vi "SaveSpeedProfileData.vi"(6 "registry":T16, 7 "data event data":T1, 8 "error in (no error)":errorcluster, 10 "pulse positions array":T9[](array[typedef]), 11 "data event config":T10) -> (0 "error out":errorcluster, 3 "data event data out":T1)   [LabVIEW 2017, in "CmsDataEventCreator.lvlib"]
uses:
  <vilib>/addons/InsightCM/Devices/Shared/Cms/CmsDataEventCreator/CmsDataEventCreator.lvlib
  <vilib>/addons/InsightCM/Devices/Shared/Cms/CmsDataEventCreator/controls/GroupRegistry.ctl
  <vilib>/addons/InsightCM/Devices/Shared/Cms/CmsDataEventCreator/controls/DataSetRegistry.ctl
  <vilib>/addons/InsightCM/Devices/Shared/Common/DataEvent/controls/DataSetType.ctl
  <vilib>/addons/InsightCM/Devices/Shared/Common/DataEventCreator/controls/Registry_Trend.ctl
  <vilib>/addons/InsightCM/Devices/Shared/Cms/CmsDataEventCreator/controls/DataEventConfig.ctl
  <vilib>/addons/InsightCM/Devices/Shared/Cms/CmsDataEventCreator/controls/AcqParams.ctl
  <vilib>/addons/InsightCM/Devices/Shared/Common/DataAccumulator/controls/AccumulationSettings.ctl
  <vilib>/addons/InsightCM/Devices/Shared/Common/DataAccumulator/controls/accumulationType.ctl
  <vilib>/addons/InsightCM/Devices/Shared/Common/DVRBuffer/controls/BufferLocation.ctl
  <vilib>/addons/PointValueMap/controls/PointMap.ctl
  <vilib>/addons/InsightCM/Utilities/Analysis/Shared/controls/PulsePositions.ctl
  <vilib>/addons/InsightCM/Devices/Shared/Common/DataEvent/controls/Event.ctl
  <vilib>/addons/InsightCM/MessageBus/Base/controls/DataEvent.ctl
  <vilib>/addons/InsightCM/MessageBus/Base/controls/KeyValuePair.ctl
  <vilib>/addons/InsightCM/Devices/Shared/Common/DataEvent/controls/DataSet.ctl
  <vilib>/addons/InsightCM/MessageBus/Base/controls/DataSetMetadata.ctl
  <vilib>/addons/InsightCM/MessageBus/Base/controls/TrendPoint.ctl
  <vilib>/addons/InsightCM/MessageBus/Base/controls/TrendAlarmUpdate.ctl
  <vilib>/addons/InsightCM/MessageBus/Base/controls/TrendAlarmTransition.ctl
  <vilib>/addons/PointValueMap/PointValueMap.lvlib
  <vilib>/addons/InsightCM/Devices/Shared/Common/DataEvent/DataEvent.lvlib
  <vilib>/addons/InsightCM/Devices/Shared/Common/DataEventCreator/DataEventCreator.lvlib
  <vilib>/addons/InsightCM/Devices/Shared/Common/DataAccumulator/DataAccumulator.lvlib
  <vilib>/addons/InsightCM/Devices/Shared/Common/DVRBuffer/DVRBuffer.lvlib
  <vilib>/addons/InsightCM/Utilities/Analysis/Shared/AnalysisHelper.lvlib
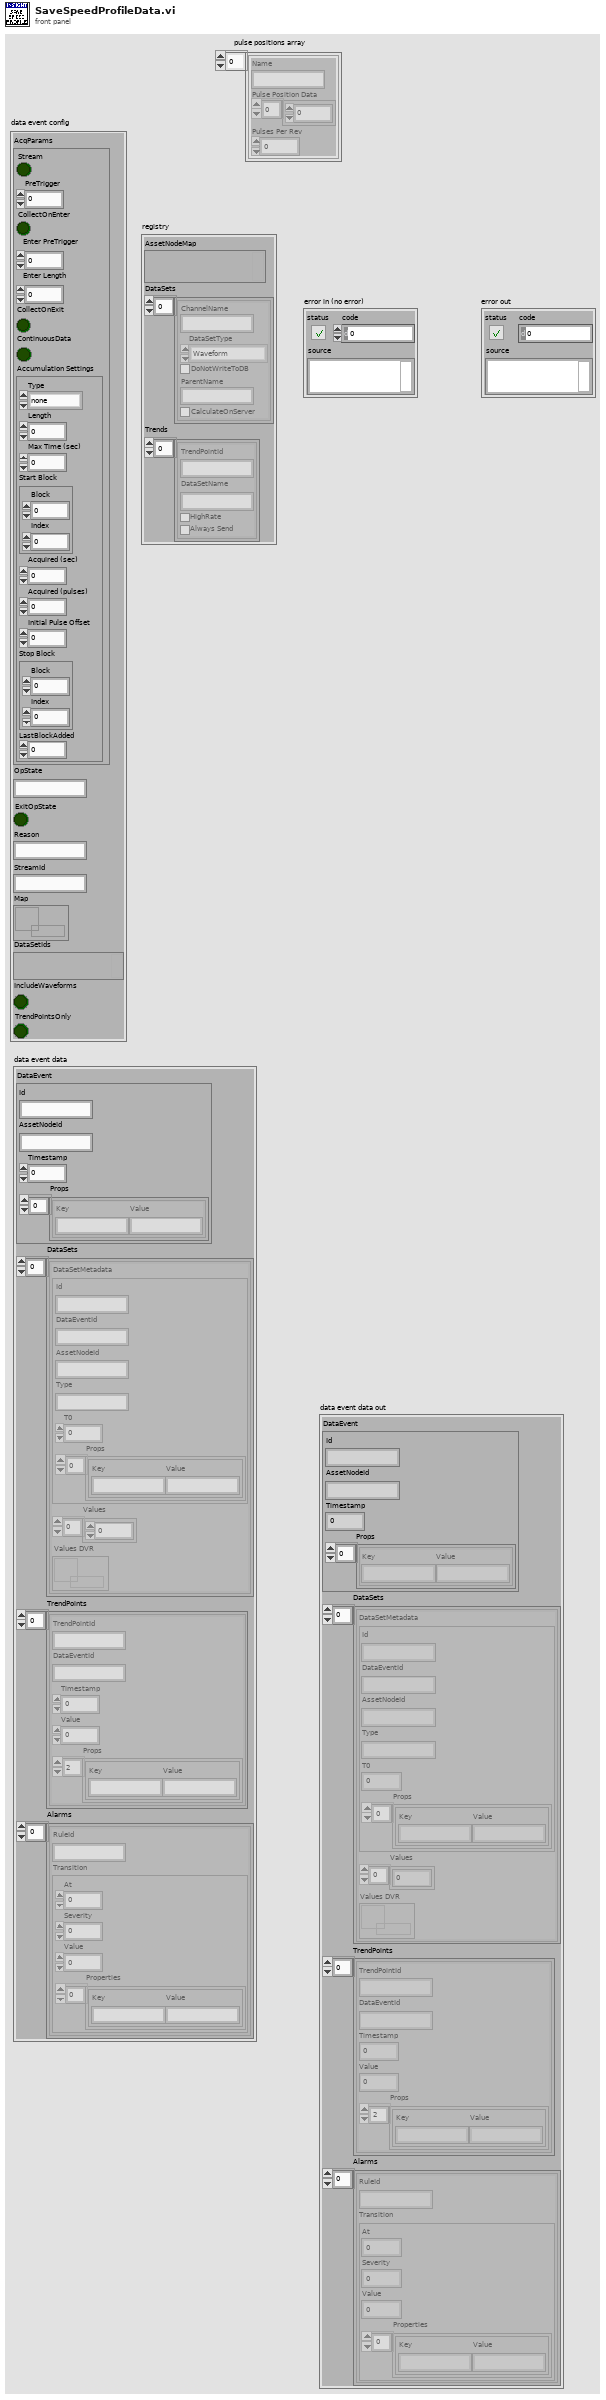
[diagram p1: front panel]
types:
  T1 = typedef "DataEvent.lvlib/Event.ctl" = cluster{"DataEvent":T2, "DataSets":T4[], "TrendPoints":T6[], "Alarms":T7[]}
  T2 = typedef "DataEvent.ctl" = cluster{"Id":string, "AssetNodeId":string, "Timestamp":i64, "Props":T3[]}
  T3 = typedef "KeyValuePair.ctl" = cluster{"Key":string, "Value":string}
  T4 = typedef "DataEvent.lvlib/DataSet.ctl" = cluster{"DataSetMetadata":T5, "Values":sgl[], "Values DVR":refnum<data-value>}
  T5 = typedef "DataSetMetadata.ctl" = cluster{"Id":string, "DataEventId":string, "AssetNodeId":string, "Type":string, "T0":i64, "Props":T3[]}
  T6 = typedef "TrendPoint.ctl" = cluster{"TrendPointId":string, "DataEventId":string, "Timestamp":i64, "Value":dbl, "Props":T3[]}
  T7 = typedef "TrendAlarmUpdate.ctl" = cluster{"RuleId":string, "Transition":T8}
  T8 = typedef "TrendAlarmTransition.ctl" = cluster{"At":i64, "Severity":i32, "Value":dbl, "Properties":T3[]}
  T9 = typedef "AnalysisHelper.lvlib/PulsePositions.ctl" = cluster{"Name":string, "Pulse Position Data":dbl[], "Pulses Per Rev":i32}
  T10 = typedef "CmsDataEventCreator.lvlib/DataEventConfig.ctl" = cluster{"AcqParams":T11, "OpState":string, "ExitOpState":bool, "Reason":string, "StreamId":string, "Map":T15, "DataSetIds":variant, "IncludeWaveforms":bool, "TrendPointsOnly":bool}
  T11 = typedef "CmsDataEventCreator.lvlib/AcqParams.ctl" = cluster{"Stream":bool, "PreTrigger":i32, "CollectOnEnter":bool, "Enter PreTrigger":i32, "Enter Length":dbl, "CollectOnExit":bool, "ContinuousData":bool, "Accumulation Settings":T12}
  T12 = typedef "DataAccumulator.lvlib/AccumulationSettings.ctl" = cluster{"Type":T13, "Length":dbl, "Max Time (sec)":dbl, "Start Block":T14, "Acquired (sec)":dbl, "Acquired (pulses)":i32, "Initial Pulse Offset":dbl, "Stop Block":T14, "LastBlockAdded":u32}
  T13 = typedef "DataAccumulator.lvlib/accumulationType.ctl" = enum16{"none", "seconds", "revolutions"}
  T14 = typedef "DVRBuffer.lvlib/BufferLocation.ctl" = cluster{"Block":u32, "Index":i32}
  T15 = typedef "PointValueMap.lvlib/PointMap.ctl" = refnum<data-value>
  T16 = typedef "CmsDataEventCreator.lvlib/GroupRegistry.ctl" = cluster{"AssetNodeMap":variant, "DataSets":T17[], "Trends":T19[]}
  T17 = typedef "CmsDataEventCreator.lvlib/DataSetRegistry.ctl" = cluster{"ChannelName":string, "DataSetType":T18, "DoNotWriteToDB":bool, "ParentName":string, "CalculateOnServer":bool}
  T18 = typedef "DataEvent.lvlib/DataSetType.ctl" = enum16{"Waveform", "SpeedProfile", "ThermalImage", "EmsaSweep"}
  T19 = typedef "DataEventCreator.lvlib/Registry_Trend.ctl" = cluster{"TrendPointId":string, "DataSetName":string, "HighRate":bool, "Always Send":bool}
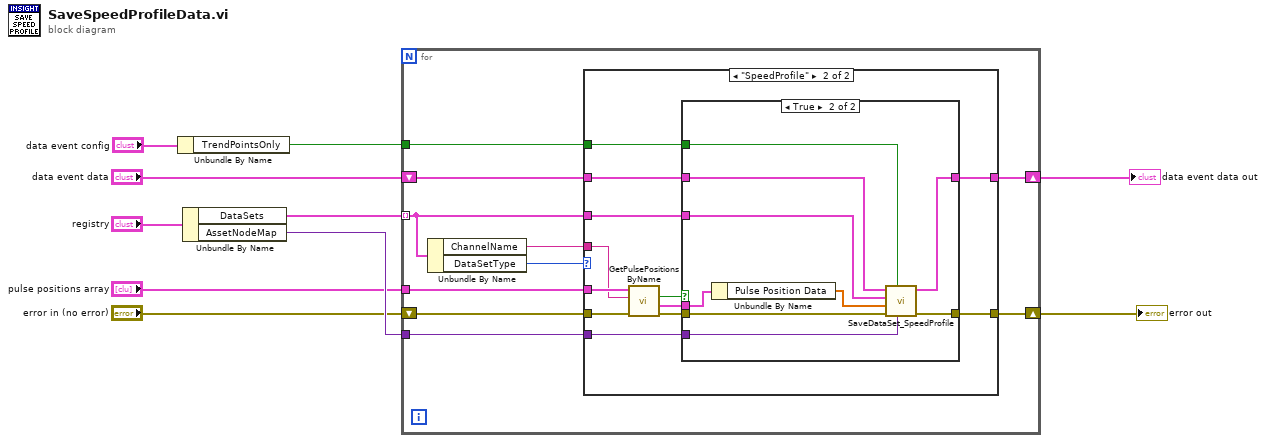
[diagram p0: block diagram]
diagram:
  n1 = Unbundle By Name("data event config") -> ("TrendPointsOnly"=w3:bool)
  n2 = Unbundle By Name("registry") -> ("DataSets"=w9:T17[], "AssetNodeMap"=w6:variant)
  n3 = for {
    tunnel: w9 -> [w13] mode=indexing
    shift-right: [w20] -> w8
    shift-left: "error in (no error)" -> [w19]
    shift-right: [w16] -> w1
    shift-left: "data event data" -> [w18]
    tunnel: "pulse positions array" -> [w15]
    tunnel: w6 -> [w12]
    tunnel: w3 -> [w11]
    n4 = Unbundle By Name(w13) -> ("ChannelName"=w17:string, "DataSetType"=w14:T18)
    n5 = case shown="\"SpeedProfile\"" w14 {
      tunnel: [w22 w34] -> w20
      tunnel: w19 -> [w22 w33]
      tunnel: w18 -> [w21 w32]
      tunnel: w17 -> [_ w26]
      tunnel: [w21 w31] -> w16
      tunnel: w15 -> [_ w30]
      tunnel: w13 -> [_ w25]
      tunnel: w12 -> [_ w24]
      tunnel: w11 -> [_ w23]
      frame Default {
      }
      frame "SpeedProfile" {
        n6 = call <vilib>:"GetPulsePositionsByName.vi"("error in (no error)"=w33, "Channel Name"=w26, "Pulse Positions Array"=w30) -> ("error out"=w29:errorcluster, "Pulse Positions"=w28:T9, "Found?"=w27:bool)  [unwired: 5 in, 1 out]
        n7 = case shown="True" w27 {
          tunnel: [w35 w44] -> w34
          tunnel: w32 -> [w36 w43]
          tunnel: [w36 w42] -> w31
          tunnel: w29 -> [w35 w45]
          tunnel: w28 -> [_ w39]
          tunnel: w25 -> [_ w41]
          tunnel: w24 -> [_ w40]
          tunnel: w23 -> [_ w37]
          frame False {
          }
          frame True {
            n8 = Unbundle By Name(w39) -> ("Pulse Position Data"=w38:dbl[])
            n9 = call <vilib>:"SaveDataSet_SpeedProfile.vi"("AssetNodeMap"=w40, "do not write to database"=w37, "error in (no error)"=w45, "speed profile"=w38, "DataSetRegistry"=w41, "event in"=w43) -> ("error out"=w44:errorcluster, "event out"=w42:T1)  [unwired: 4 in]
          }
        }
      }
    }
  }
  "error out" <- w8
  "data event data out" <- w1
